vi "to string.vi"(8 "error in":errorcluster, 11 "configuration in":refnum<class "NISE_CEF_serializable configuration.lvclass">) -> (0 "error out":errorcluster, 1 "data":string, 2 "version":string, 3 "configuration out":refnum<class "NISE_CEF_serializable configuration.lvclass">)   [LabVIEW 2013, in "NISE_CEF_serializable configuration.lvclass"]
doc: "Provides an interface for saving a module configuration to a file or other serialized data source. It is recommended that all children of this class store data in two sets--data required for its own initialization, and any data required for parent initialization--and that each implementation uses the <b>Call Parent Method</b> primitive to serialize parent information."
uses:
  NISE_CEF_serializable configuration.lvclass
  NISE_CEF_serializable configuration.lvclass/NISE_CEF_serializable configuration.ctl
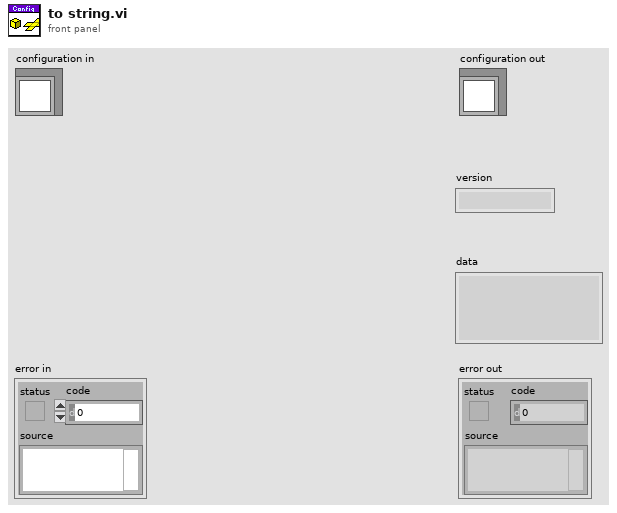
[diagram p1: front panel]
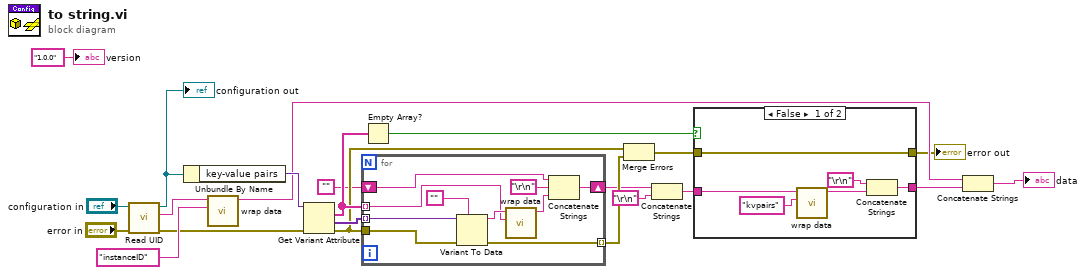
[diagram p0: block diagram]
diagram:
  n1 = call "Read UID.vi"("error in"="error in", "configuration in"="configuration in") -> ("error out"=w13:errorcluster, "instance id"=w21:string, "configuration out"=w14:refnum<class "NISE_CEF_serializable configuration.lvclass">)  [unwired: 7 in]
  "configuration out" <- w14
  n2 = Unbundle By Name(w14) -> ("key-value pairs"=w18:variant)
  n3 = call "wrap data.vi"("identifier"="instanceID" ("additional identifier"), "data to wrap"=w21) -> ("wrapped data"=w16:string)  [unwired: 9 in]
  n4 = Get Variant Attribute(Variant=w18, error in=w13) -> (names=w9:string[], values=w17:variant[], error out=w6:errorcluster)  [unwired: 2 in, 1 out]
  n5 = for {
    tunnel: w17 -> [w31] mode=indexing
    tunnel: w9 -> [w29] mode=indexing
    tunnel: [w27] -> w7 mode=indexing
    tunnel: w6 -> [w28]
    shift-right: [w24] -> w4
    shift-left: "" -> [w26]
    n6 = Variant To Data(error in=w28, type="", Variant=w31) -> (data=w30:string, error out=w27:errorcluster)
    n7 = call "wrap data.vi"("identifier"=w29, "data to wrap"=w30) -> ("wrapped data"=w23:string)  [unwired: 9 in]
    n8 = Concatenate Strings(w26, "\r\n", w23) -> (w24:string)
  }
  n9 = Empty Array?(array=w9) -> (empty?=w11:bool)
  n10 = Merge Errors(w6, w7) -> (w8:errorcluster)
  n11 = Concatenate Strings(w4, "\r\n") -> (w3:string)
  n12 = case shown="False" w11 {
    tunnel: w8 -> [w38 w39]
    tunnel: [w38 w39] -> w12
    tunnel: [w35 _] -> w10
    tunnel: w3 -> [w34 _]
    frame False {
      n13 = call "wrap data.vi"("identifier"="kvpairs" ("additional identifier"), "data to wrap"=w34) -> ("wrapped data"=w36:string)  [unwired: 9 in]
      n14 = Concatenate Strings("\r\n", w36) -> (w35:string)
    }
    frame True {
    }
  }
  "error out" <- w12
  n15 = Concatenate Strings(w16, w10) -> (→"data":string)
  "version" <- "1.0.0" ("version")
